vi "Example_AOU.vi"() -> ()   [LabVIEW 2013]
uses:
  <vilib>/Signadyne/Wave/base/waveformLoadWave.vi
panel:
  out "Waveform Memory":string[](array[string])
  in  "Stop":bool
  in  "AWG index":u32
  out "AWG queue":i32[][](array[numeric])
  in  "Run":bool
  in  "Flush AWG":bool
  in  "Queue Waveform":bool
  in  "AWG":u32
  in  "Waveform number":u32
  out "errorOut":errorcluster
  in  "Flush Waveforms":bool
  in  "Close":bool
  in  "Load Waveform":bool
  in  "Prescaler":u32
  in  "Cycles":u32
  in  "Start Delay":u32
  in  "Trigger Mode":T1(ring)
  in  "Waveform number":u32
  in  "Frequency":dbl
  in  "Amplitude":dbl
  in  "Deviation Gain":u32
  in  "Modulation Type":T2(ring)
  in  "Waveform Path":path
  in  "Wave Shape":T3(ring)
  in  "nSlot":i32=7
  in  "nChassis":i32=1
  in  "partNumber":string="SD-PXE-AOU-H0002-128"
  in  "Channel":u32
  # "Module Under Test"
  # "Modulation"
  # "AWG queue"
  # "Waveform Memory"
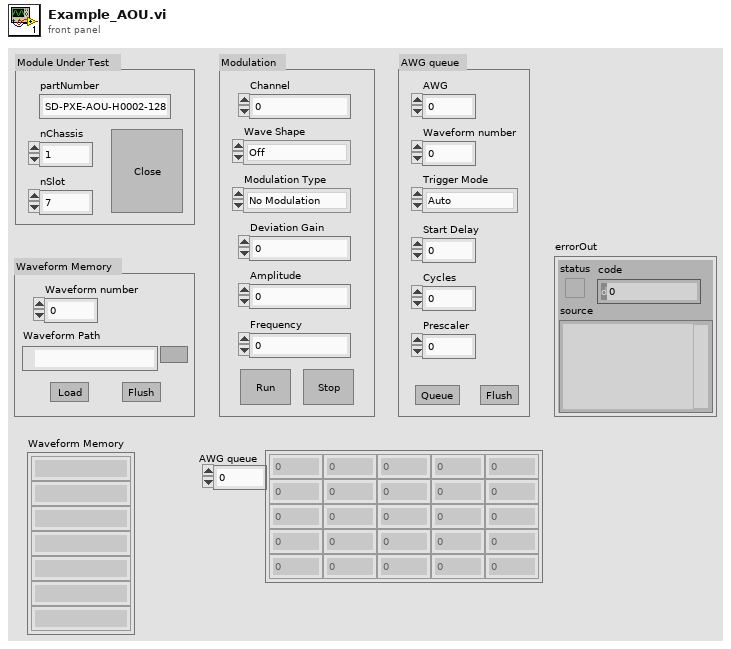
[diagram p1: front panel]
types:
  T1 = enum32{"Auto", "VI/HVI Trigger", "External Trigger"}
  T2 = enum32{"No Modulation", "Amplitude Modulation", "Offet Modulation", "Amplitude & Offset Modulation"}
  T3 = enum32{"Off", "Sinusoidal", "Triangular", "Sawtooth", "Square", "DC", "Arbitrary Waveform"}
  T4 = cluster{"initialized array":i32[][], "initialized array":i32[][], "initialized array":i32[][], "initialized array":i32[][]}
  T5 = cluster{"Array":i32[][], "Array":i32[][], "Array":i32[][], "Array":i32[][]}
  T6 = cluster{"Array[0]":i32, "Array[1]":i32, "Array[2]":i32, "Array[3]":i32, "Array[4]":i32, "Array[5]":i32, "Array[6]":i32, "Array[7]":i32, "Array[8]":i32}
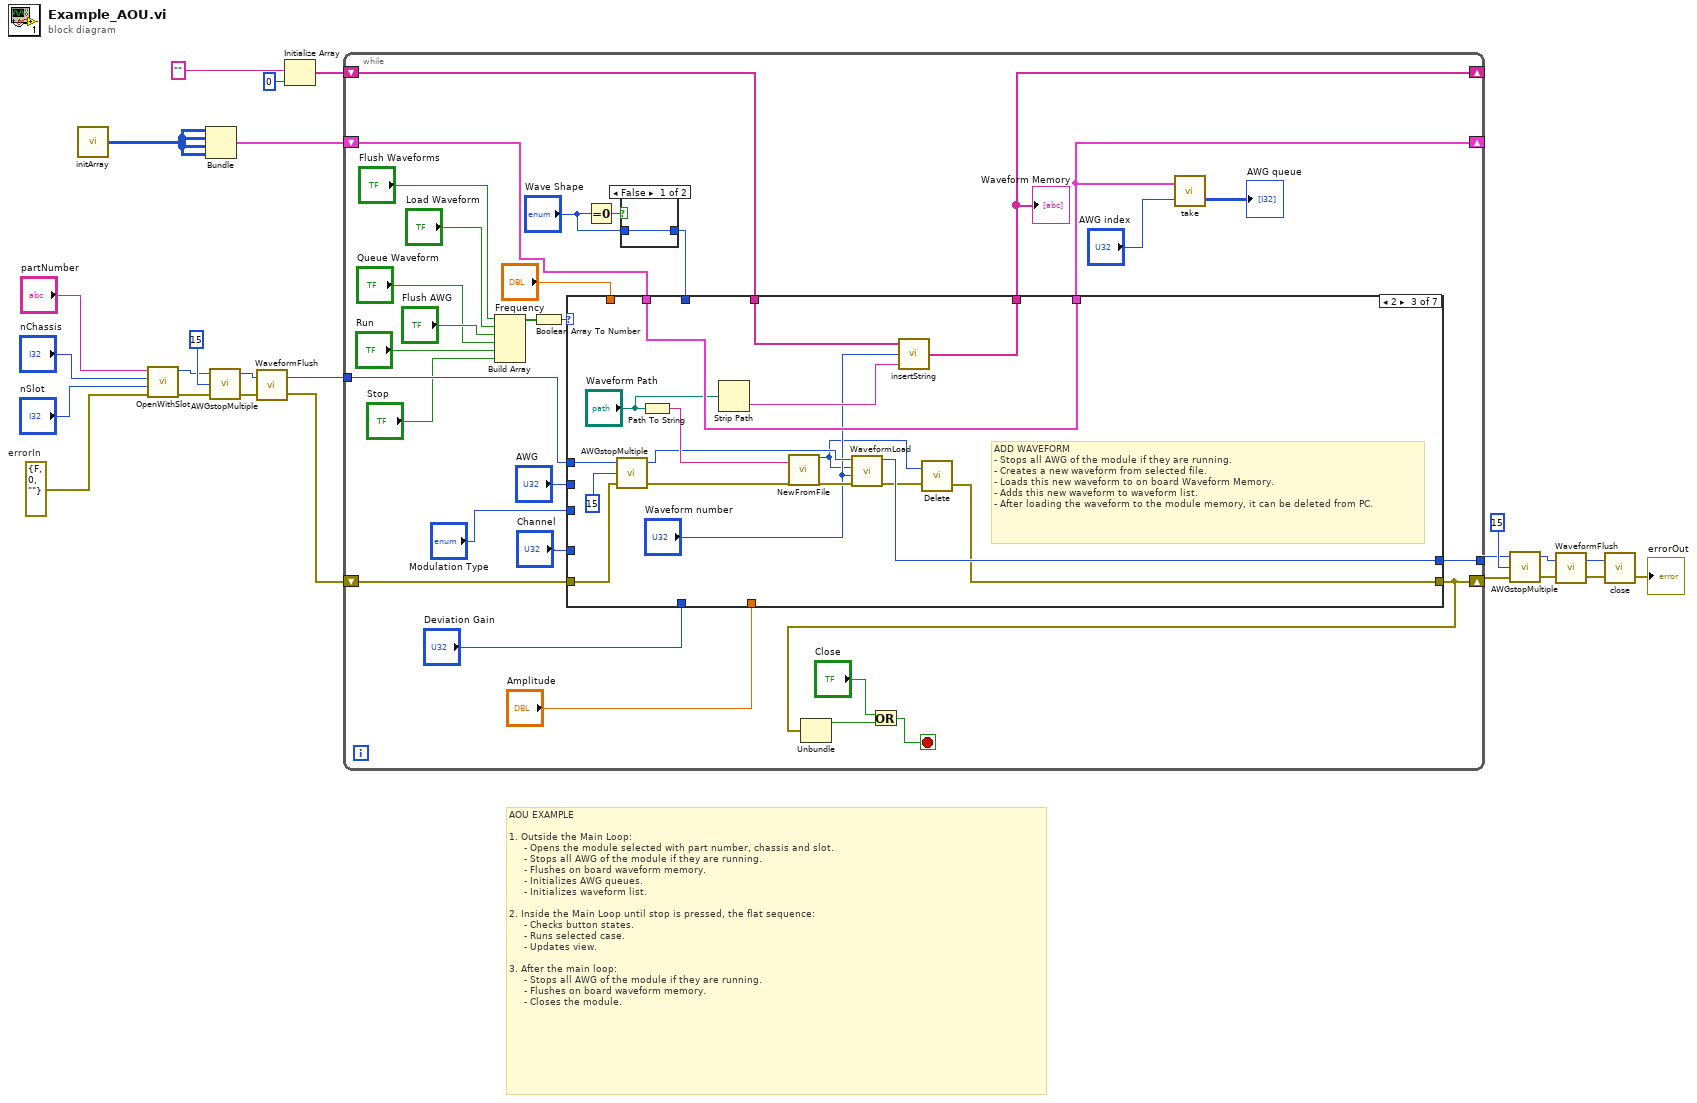
[diagram p0: block diagram]
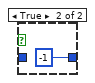
[diagram p2: hidden frame]
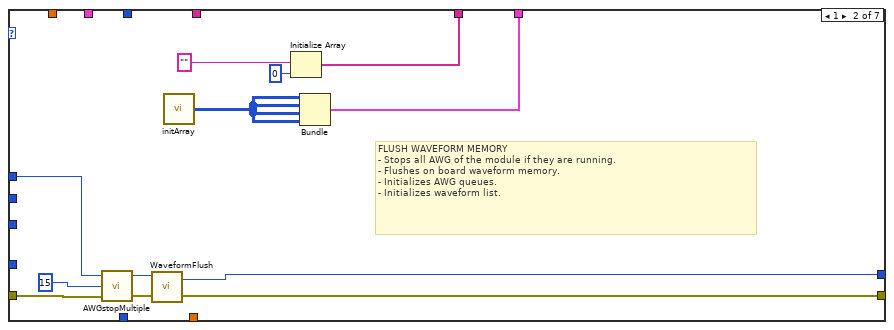
[diagram p4: hidden frame]
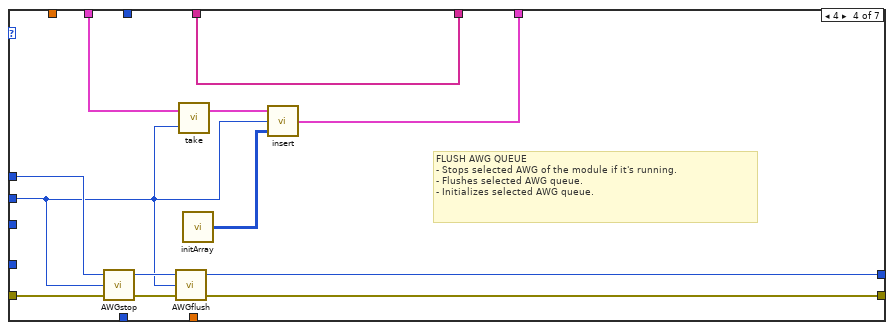
[diagram p5: hidden frame]
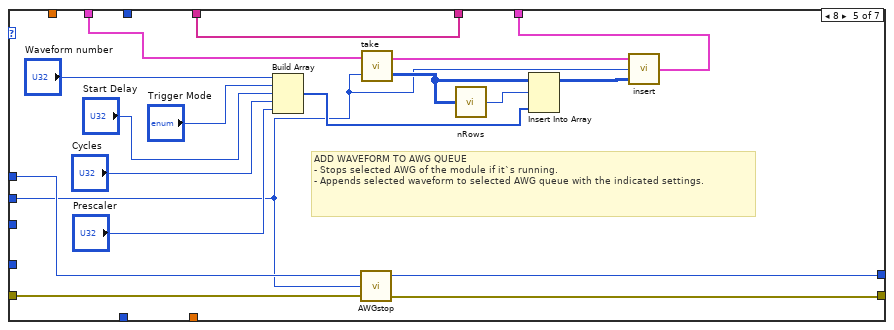
[diagram p6: hidden frame]
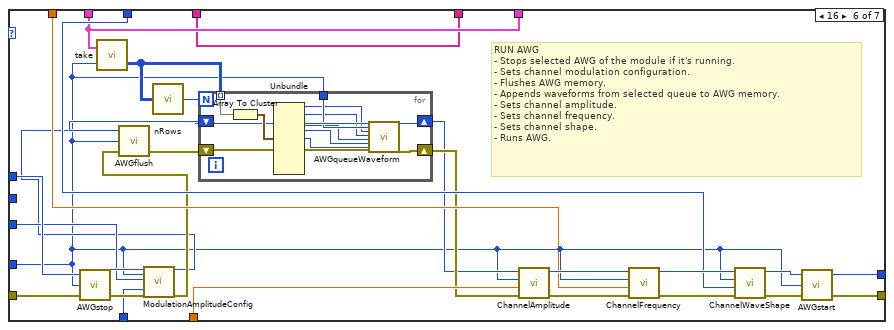
[diagram p7: hidden frame]
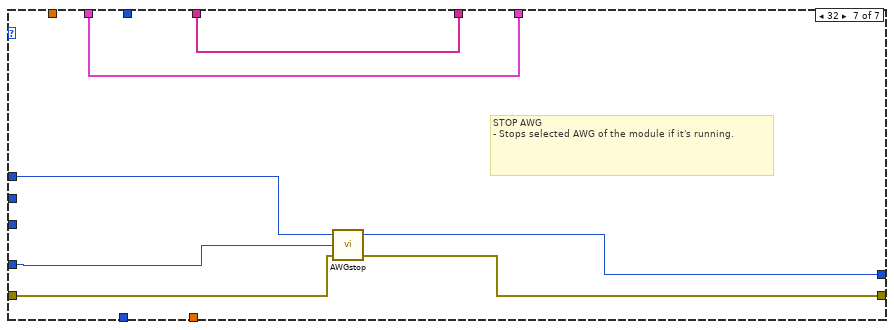
[diagram p8: hidden frame]
diagram:
  w6 = errorcluster {"status"=FALSE, "code"=0, "source"=""}  # errorIn
  # "AOU EXAMPLE\n\n1. Outside the Main Loop:\n     - Opens the module selected with part number, chassis and slot.\n     - Stops all AWG of the module if they are running.\n     - Flushes on board waveform memory.\n     - Initializes AWG queues.\n     - Initializes waveform list.\n\n2. Inside the Main Loop until stop is pressed, the flat sequence:\n     - Checks button states.\n     - Runs selected case.\n     - Updates view.\n\n3. After the main loop:\n     - Stops all AWG of the module if they are running.\n     - Flushes on board waveform memory.\n     - Closes the module."
  n1 = call "initArray.vi"() -> ("initialized array"=w4:i32[][])
  n2 = call <vilib>:"OpenWithSlot.vi"("errorIn"=w6, "nSlot"="nSlot", "nChassis"="nChassis", "partNumber"="partNumber") -> ("errorOut"=w8:errorcluster, "moduleID"=w9:i32)  [unwired: 2 in]
  n3 = Bundle("initialized array"=w4, "initialized array"=w4, "initialized array"=w4, "initialized array"=w4) -> (w5:T4)  [unwired: 1 in]
  n4 = call <vilib>:"AWGstopMultiple.vi"("errorIn"=w8, "AWGmask"=15, "moduleID"=w9) -> ("errorOut"=w11:errorcluster, "moduleIDOut"=w10:i32)  [unwired: 1 in]
  n5 = call <vilib>:"WaveformFlush.vi"("errorIn"=w11, "moduleID"=w10) -> ("errorOut"=w21:errorcluster, "moduleIDOut"=w22:i32)
  n6 = Initialize Array("", 0 ("dimension size")) -> (w3:string[])
  n7 = while {
    tunnel: w22 -> [w50]
    shift-right: [w35] -> w15
    shift-left: w21 -> [w54]
    tunnel: [w49] -> w16
    shift-right: [w28] -> _
    shift-left: w5 -> [w31]
    shift-right: [w25] -> _
    shift-left: w3 -> [w26]
    stop <- w33 stop-if-true
    n8 = Build Array("Flush Waveforms", "Load Waveform", "Flush AWG", "Queue Waveform", "Run", "Stop") -> (w51:bool[])
    n9 = Boolean Array To Number(Boolean array=w51) -> (number=w53:u32)
    n10 = Equal To 0?(x="Wave Shape") -> (x = 0?=w37:bool)
    n11 = case shown="False" w37 {
      tunnel: "Wave Shape" -> [w55 _]
      tunnel: [w55 -1] -> w36
      frame False {
      }
      frame True {
      }
    }
    n12 = case shown="2" w53 {
      tunnel: w54 -> [w60 w68 w85 w99 w119 w147 w165]
      tunnel: [w60 w72 w74 w96 w112 w135 w163] -> w35
      tunnel: w50 -> [w59 w67 w83 w97 w118 w146 w164]
      tunnel: [w59 w71 w87 w101 w111 w134 w162] -> w49
      tunnel: "AWG" -> [_ _ _ w90 w102 _ _]
      tunnel: "Channel" -> [_ _ _ _ _ w120 w160]
      tunnel: "Deviation Gain" -> [_ _ _ _ _ w144 _]
      tunnel: "Modulation Type" -> [_ _ _ _ _ w136 _]
      tunnel: "Amplitude" -> [_ _ _ _ _ w142 _]
      tunnel: "Frequency" -> [_ _ _ _ _ w139 _]
      tunnel: w36 -> [_ _ _ _ _ w131 _]
      tunnel: w31 -> [w58 _ w81 w95 w109 w124 w166]
      tunnel: [w58 w65 w81 w93 w108 w124 w166] -> w28
      tunnel: w26 -> [w57 _ w78 w91 w103 w121 w161]
      tunnel: [w57 w61 w79 w91 w103 w121 w161] -> w25
      frame 0, Default {
        # "DO NOTHING"
      }
      frame 1 {
        # "FLUSH WAVEFORM MEMORY\n- Stops all AWG of the module if they are running.\n- Flushes on board waveform memory.\n- Initializes AWG queues.\n- Initializes waveform list."
        n13 = call <vilib>:"AWGstopMultiple.vi"("errorIn"=w68, "AWGmask"=15, "moduleID"=w67) -> ("errorOut"=w70:errorcluster, "moduleIDOut"=w69:i32)  [unwired: 1 in]
        n14 = call <vilib>:"WaveformFlush.vi"("errorIn"=w70, "moduleID"=w69) -> ("errorOut"=w72:errorcluster, "moduleIDOut"=w71:i32)
        n15 = call "initArray.vi"() -> ("initialized array"=w64:i32[][])
        n16 = Initialize Array("", 0 ("dimension size")) -> (w61:string[])
        n17 = Bundle("initialized array"=w64, "initialized array"=w64, "initialized array"=w64, "initialized array"=w64) -> (w65:T4)  [unwired: 1 in]
      }
      frame 2 {
        # "ADD WAVEFORM\n- Stops all AWG of the module if they are running.\n- Creates a new waveform from selected file.\n- Loads this new waveform to on board Waveform Memory.\n- Adds this new waveform to waveform list.\n- After loading the waveform to the module memory, it can be deleted from PC."
        n18 = call <vilib>:"AWGstopMultiple.vi"("errorIn"=w85, "AWGmask"=15, "moduleID"=w83) -> ("errorOut"=w84:errorcluster, "moduleIDOut"=w82:i32)  [unwired: 1 in]
        n19 = Path To String(path="Waveform Path") -> (string=w89:string)
        n20 = Strip Path(path="Waveform Path") -> (name=w77:string)  [unwired: 1 out]
        n21 = call <vilib>:"NewFromFile.vi"("waveformFile"=w89, "errorIn"=w84) -> ("waveformID"=w73:i32, "errorOut"=w88:errorcluster)  [unwired: 16 in]
        n22 = call-poly <vilib>:"WaveformLoad.vi"("errorIn"=w88, "waveformNumber"="Waveform number", "waveformID"=w73, "moduleID"=w82) -> ("errorOut"=w76:errorcluster, "moduleIDOut"=w87:i32)  [unwired: 3 in, 1 out]
        n23 = call "insertString.vi"("input"=w77, "index"="Waveform number", "array"=w78) -> ("output array"=w79:string[])
        n24 = call <vilib>:"Delete.vi"("errorIn"=w76, "waveformID"=w73) -> ("errorOut"=w74:errorcluster)  [unwired: 1 in]
      }
      frame 4 {
        # "FLUSH AWG QUEUE\n- Stops selected AWG of the module if it's running.\n- Flushes selected AWG queue.\n- Initializes selected AWG queue."
        n25 = call <vilib>:"AWGstop.vi"("errorIn"=w99, "nAWG"=w90, "moduleID"=w97) -> ("errorOut"=w100:errorcluster, "moduleIDOut"=w98:i32)  [unwired: 1 in]
        n26 = call <vilib>:"AWGflush.vi"("errorIn"=w100, "nAWG"=w90, "moduleID"=w98) -> ("errorOut"=w96:errorcluster, "moduleIDOut"=w101:i32)  [unwired: 1 in]
        n27 = call "take.vi"("AWG index"=w90, "cluster"=w95) -> ("output cluster"=w94:cluster{i32[][], i32[][], i32[][]})  [unwired: 1 out]
        n28 = call "initArray.vi"() -> ("initialized array"=w92:i32[][])
        n29 = call "insert.vi"("Array"=w92, "AWG index"=w90, "cluster"=w94) -> ("output cluster"=w93:T5)
      }
      frame 8 {
        # "ADD WAVEFORM TO AWG QUEUE\n- Stops selected AWG of the module if it`s running.\n- Appends selected waveform to selected AWG queue with the indicated settings."
        n30 = Build Array("Waveform number", "Trigger Mode", "Start Delay", "Cycles", "Prescaler") -> (w110:u32[])
        n31 = call <vilib>:"AWGstop.vi"("errorIn"=w119, "nAWG"=w102, "moduleID"=w118) -> ("errorOut"=w112:errorcluster, "moduleIDOut"=w111:i32)  [unwired: 1 in]
        n32 = call "take.vi"("AWG index"=w102, "cluster"=w109) -> ("Array"=w104:i32[][], "output cluster"=w106:cluster{i32[][], i32[][], i32[][]})
        n33 = call "nRows.vi"("array"=w104) -> ("Numeric"=w105:i32)
        n34 = Insert Into Array(array=w104, index (row)=w105, new element=w110) -> (w107:i32[][])  [unwired: 1 in]
        n35 = call "insert.vi"("Array"=w107, "AWG index"=w102, "cluster"=w106) -> ("output cluster"=w108:T5)
      }
      frame 16 {
        # "RUN AWG\n- Stops selected AWG of the module if it's running.\n- Sets channel modulation configuration.\n- Flushes AWG memory.\n- Appends waveforms from selected queue to AWG memory.\n- Sets channel amplitude.\n- Sets channel frequency.\n- Sets channel shape.\n- Runs AWG."
        n36 = call <vilib>:"AWGstop.vi"("errorIn"=w147, "nAWG"=w120, "moduleID"=w146) -> ("errorOut"=w145:errorcluster, "moduleIDOut"=w143:i32)  [unwired: 1 in]
        n37 = call "take.vi"("AWG index"=w120, "cluster"=w124) -> ("Array"=w122:i32[][])  [unwired: 1 out]
        n38 = call <vilib>:"ModulationAmplitudeConfig.vi"("moduleID"=w143, "nChannel"=w120, "modulationType"=w136, "deviationGain"=w144, "errorIn"=w145) -> ("moduleIDOut"=w125:i64, "errorOut"=w128:errorcluster)  [unwired: 13 in]
        n39 = call <vilib>:"AWGflush.vi"("errorIn"=w128, "nAWG"=w120, "moduleID"=w125) -> ("errorOut"=w127:errorcluster, "moduleIDOut"=w126:i32)  [unwired: 1 in]
        n40 = call "nRows.vi"("array"=w122) -> ("Numeric"=w123:i32)
        n41 = for {
          N: w123 -> [_]
          tunnel: w122 -> [w159] mode=indexing
          shift-right: [w155] -> w129
          shift-left: w126 -> [w156]
          shift-right: [w154] -> w130
          shift-left: w127 -> [w157]
          tunnel: w120 -> [w153]
          n42 = Array To Cluster(array=w159) -> (cluster=w158:T6)
          n43 = Unbundle(w158) -> ("Array[0]"=w152:i32, "Array[1]"=w151:i32, "Array[2]"=w150:i32, "Array[3]"=w149:i32, "Array[4]"=w148:i32)  [unwired: 4 out]
          n44 = call <vilib>:"AWGqueueWaveform.vi"("moduleID"=w156, "nAWG"=w153, "waveformNumber"=w152, "triggerMode"=w151, "startDelay"=w150, "cycles"=w149, "prescaler"=w148, "errorIn"=w157) -> ("moduleIDOut"=w155:i32, "errorOut"=w154:errorcluster)  [unwired: 18 in]
        }
        n45 = call <vilib>:"ChannelAmplitude.vi"("errorIn"=w130, "amplitude"=w142, "nChannel"=w120, "moduleID"=w129) -> ("errorOut"=w141:errorcluster, "moduleIDOut"=w140:i32)  [unwired: 2 in]
        n46 = call <vilib>:"ChannelFrequency.vi"("errorIn"=w141, "frequency"=w139, "nChannel"=w120, "moduleID"=w140) -> ("errorOut"=w137:errorcluster, "moduleIDOut"=w138:i32)  [unwired: 2 in]
        n47 = call <vilib>:"ChannelWaveShape.vi"("errorIn"=w137, "waveShape"=w131, "nChannel"=w120, "moduleID"=w138) -> ("errorOut"=w133:errorcluster, "moduleIDOut"=w132:i32)  [unwired: 2 in]
        n48 = call <vilib>:"AWGstart.vi"("errorIn"=w133, "nAWG"=w120, "moduleID"=w132) -> ("errorOut"=w135:errorcluster, "moduleIDOut"=w134:i32)  [unwired: 1 in]
      }
      frame 32 {
        # "STOP AWG\n- Stops selected AWG of the module if it's running."
        n49 = call <vilib>:"AWGstop.vi"("errorIn"=w165, "nAWG"=w160, "moduleID"=w164) -> ("errorOut"=w163:errorcluster, "moduleIDOut"=w162:i32)  [unwired: 1 in]
      }
    }
    "Waveform Memory" <- w25
    n50 = Unbundle(w35) -> ("status"=w34:bool)  [unwired: 2 out]
    n51 = Or(x="Close", y=w34) -> (x .or. y?=w33:bool)
    n52 = call "take.vi"("AWG index"="AWG index", "cluster"=w28) -> ("Array"=→"AWG queue":i32[][])  [unwired: 1 out]
  }
  n53 = call <vilib>:"AWGstopMultiple.vi"("errorIn"=w15, "AWGmask"=15, "moduleID"=w16) -> ("errorOut"=w14:errorcluster, "moduleIDOut"=w13:i32)  [unwired: 1 in]
  n54 = call <vilib>:"WaveformFlush.vi"("errorIn"=w14, "moduleID"=w13) -> ("errorOut"=w19:errorcluster, "moduleIDOut"=w18:i32)
  n55 = call <vilib>:"close.vi"("errorIn"=w19, "moduleID"=w18) -> ("errorOut"=→"errorOut":errorcluster)  [unwired: 1 in]
